vi "JAVA_DriveSignal.vi"   [LabVIEW 2016]
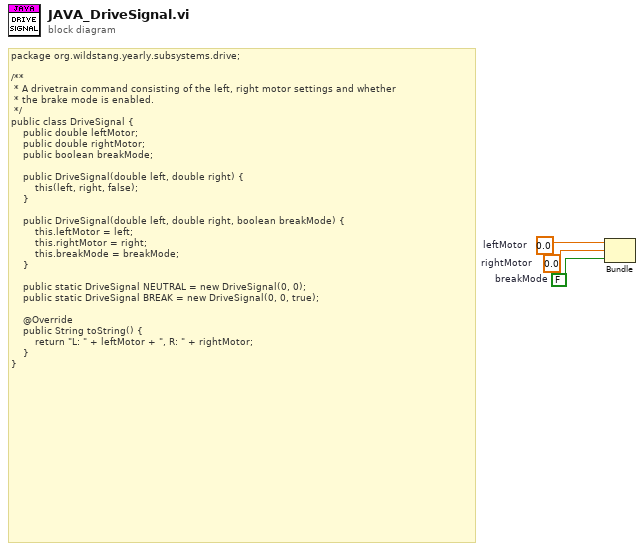
[diagram p0: block diagram]
diagram:
  w1 = FALSE  # breakMode
  w2 = 0.0  # rightMotor
  w3 = 0.0  # leftMotor
  # "package org.wildstang.yearly.subsystems.drive;\n\n/**\n * A drivetrain command consisting of the left, right motor settings and whether\n * the brake mode is enabled.\n */\npublic class DriveSignal {\n    public double leftMotor;\n    public double rightMotor;\n    public boolean breakMode;\n\n    public DriveSignal(double left, double right) {\n        this(left, right, false);\n    }\n\n    public DriveSignal(double left, double right, boolean breakMode) {\n        this.leftMotor = left;\n        this.rightMotor = right;\n        this.breakMode = breakMode;\n    }\n\n    public static DriveSignal NEUTRAL = new DriveSignal(0, 0);\n    public static DriveSignal BREAK = new DriveSignal(0, 0, true);\n\n    @Override\n    public String toString() {\n        return \"L: \" + leftMotor + \", R: \" + rightMotor;\n    }\n}"
  n1 = Bundle("leftMotor"=w3, "rightMotor"=w2, "breakMode"=w1) -> ()  [unwired: 1 in, 1 out]
